vi "Read Cursors.vi"(0 "VISA Resource Name":refnum<visa-resource-name>, 11 "error in (no error)":errorcluster) -> (1 "horiz pos 1":dbl format="%.7f", 2 "horiz pos 2":dbl format="%.7f", 3 "horiz delta":dbl format="%.7f", 4 "VISA Resource Name Out":refnum<visa-resource-name>, 6 "horiz units":i32(ring) items=["Volts", "Amps", "Amp^2", "Amp/Volt", "Volt/Amp", "Volts^2", "Watt", "%", "IRE"], 10 "vert units":i32(ring) items=["Seconds", "Hertz", "Percent", "Degrees"], 12 "vert pos 1":dbl format="%.7f", 13 "vert pos 2":dbl format="%.7f", 14 "vert delta":dbl format="%.7f", 15 "error out":errorcluster)   [LabVIEW 2010, in "Tektronix TDS 3000 Series.lvlib"]
doc: "This VI returns the positions, delta values and units of the horizontal and vertical cursors on the scope."
uses:
  <instrlib>/Tektronix TDS 3000 Series/Tektronix TDS 3000 Series.lvlib
  <vilib>/Utility/error.llb/whitespace.ctl
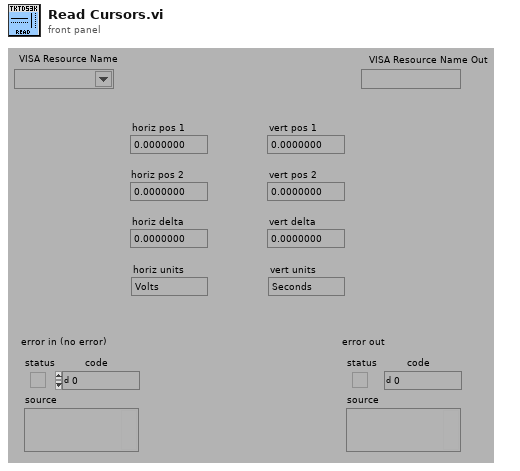
[diagram p1: front panel]
types:
  T1 = typedef "whitespace.ctl" = u16
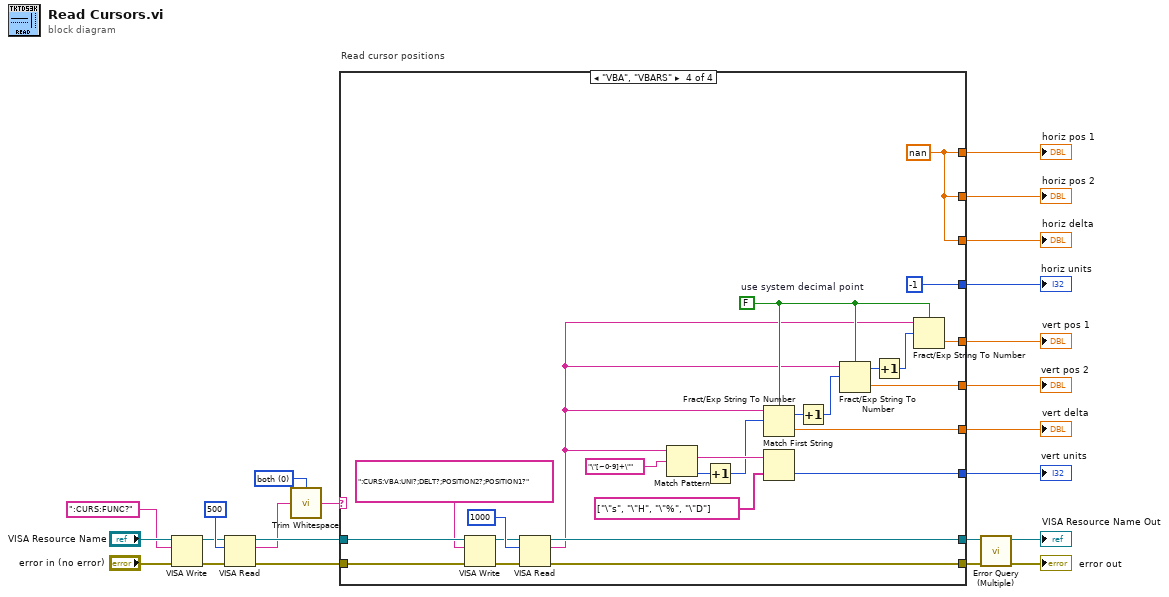
[diagram p0: block diagram]
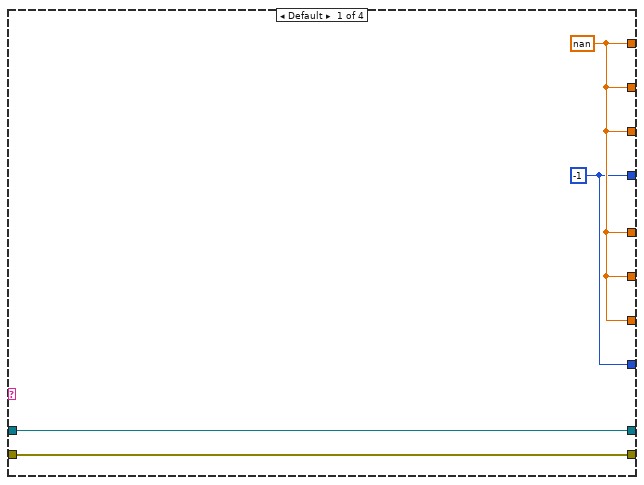
[diagram p2: hidden frame]
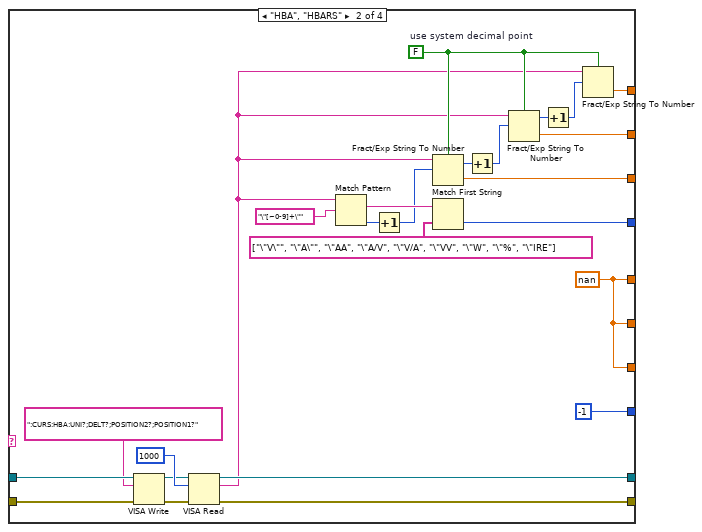
[diagram p3: hidden frame]
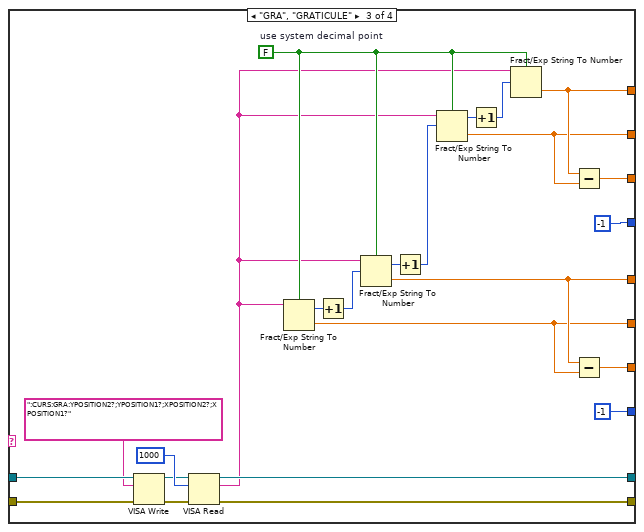
[diagram p4: hidden frame]
diagram:
  w7 = T1 0 items=["both", "start of string", "end of string"] ("location (both)")
  # "Read cursor positions"
  n1 = VISA Write(VISA resource name="VISA Resource Name", write buffer=":CURS:FUNC?", error in (no error)="error in (no error)") -> (VISA resource name out=w19:refnum<visa-resource-name>, error out=w18:errorcluster)  [unwired: 1 out]
  n2 = VISA Read(VISA resource name=w19, byte count=u32 500, error in (no error)=w18) -> (VISA resource name out=w11:refnum<visa-resource-name>, read buffer=w8:string, error out=w10:errorcluster)  [unwired: 1 out]
  n3 = call <vilib>:"Trim Whitespace.vi"("string"=w8, "location (both)"=w7) -> ("trimmed string"=w9:string)
  n4 = case shown="\"VBA\", \"VBARS\"" w9 {
    tunnel: [w25 w40 w58 w98] -> w17
    tunnel: [w25 w39 w57 w98] -> w16
    tunnel: [w25 w38 w56 w98] -> w15
    tunnel: [w25 w41 w54 w80] -> w14
    tunnel: [w25 w41 w53 w81] -> w13
    tunnel: [w25 w41 w55 w82] -> w12
    tunnel: [w26 w52 w76 w101] -> w3
    tunnel: [w27 w51 w75 w100] -> w4
    tunnel: w11 -> [w27 w48 w73 w97]
    tunnel: w10 -> [w26 w45 w70 w94]
    tunnel: [w24 -1 ("index") -1 ("index") w83] -> w6
    tunnel: [w24 w37 -1 ("index") -1 ("index")] -> w5
    frame Default {
      w24 = -1 ("index")
      w25 = nan
    }
    frame "HBA", "HBARS" {
      w49 = FALSE  # use system decimal point
      w41 = nan
      n5 = VISA Write(VISA resource name=w48, write buffer=":CURS:HBA:UNI?;DELT?;POSITION2?;POSITION1?", error in (no error)=w45) -> (VISA resource name out=w47:refnum<visa-resource-name>, error out=w46:errorcluster)  [unwired: 1 out]
      n6 = VISA Read(VISA resource name=w47, byte count=u32 1000, error in (no error)=w46) -> (VISA resource name out=w51:refnum<visa-resource-name>, read buffer=w36:string, error out=w52:errorcluster)  [unwired: 1 out]
      n7 = Match Pattern(string=w36, regular expression="\"[~0-9]+\"") -> (match substring=w31:string, offset past match=w30:i32)  [unwired: 1 in, 2 out]
      n8 = Increment(x=w30) -> (x+1=w29:i32)
      n9 = Fract/Exp String To Number(use system decimal point (T)=w49, string=w36, offset=w29) -> (offset past number=w35:i32, number=w38:dbl)  [unwired: 1 in]
      n10 = Match First String(2:string[] ["\"V\"", "\"A\"", "\"AA", "\"A/V", "\"V/A", "\"VV", "\"W", "\"%", "\"IRE"], 3:w31) -> (0:w37:i32)  [unwired: 1 out]
      n11 = Increment(x=w35) -> (x+1=w34:i32)
      n12 = Fract/Exp String To Number(use system decimal point (T)=w49, string=w36, offset=w34) -> (offset past number=w33:i32, number=w39:dbl)  [unwired: 1 in]
      n13 = Increment(x=w33) -> (x+1=w32:i32)
      n14 = Fract/Exp String To Number(use system decimal point (T)=w49, string=w36, offset=w32) -> (number=w40:dbl)  [unwired: 1 in, 1 out]
    }
    frame "GRA", "GRATICULE" {
      w60 = FALSE  # use system decimal point
      n15 = VISA Write(VISA resource name=w73, write buffer=":CURS:GRA:YPOSITION2?;YPOSITION1?;XPOSITION2?;XPOSITION1?", error in (no error)=w70) -> (VISA resource name out=w72:refnum<visa-resource-name>, error out=w71:errorcluster)  [unwired: 1 out]
      n16 = VISA Read(VISA resource name=w72, byte count=u32 1000, error in (no error)=w71) -> (VISA resource name out=w75:refnum<visa-resource-name>, read buffer=w59:string, error out=w76:errorcluster)  [unwired: 1 out]
      n17 = Fract/Exp String To Number(use system decimal point (T)=w60, string=w59) -> (offset past number=w62:i32, number=w53:dbl)  [unwired: 2 in]
      n18 = Increment(x=w62) -> (x+1=w61:i32)
      n19 = Fract/Exp String To Number(use system decimal point (T)=w60, string=w59, offset=w61) -> (offset past number=w66:i32, number=w54:dbl)  [unwired: 1 in]
      n20 = Increment(x=w66) -> (x+1=w65:i32)
      n21 = Fract/Exp String To Number(use system decimal point (T)=w60, string=w59, offset=w65) -> (offset past number=w64:i32, number=w57:dbl)  [unwired: 1 in]
      n22 = Increment(x=w64) -> (x+1=w63:i32)
      n23 = Fract/Exp String To Number(use system decimal point (T)=w60, string=w59, offset=w63) -> (number=w58:dbl)  [unwired: 1 in, 1 out]
      n24 = Subtract(x=w58, y=w57) -> (x-y=w56:dbl)
      n25 = Subtract(x=w54, y=w53) -> (x-y=w55:dbl)
    }
    frame "VBA", "VBARS" {
      w91 = FALSE  # use system decimal point
      w98 = nan
      n26 = VISA Write(VISA resource name=w97, write buffer=":CURS:VBA:UNI?;DELT?;POSITION2?;POSITION1?", error in (no error)=w94) -> (VISA resource name out=w96:refnum<visa-resource-name>, error out=w95:errorcluster)  [unwired: 1 out]
      n27 = VISA Read(VISA resource name=w96, byte count=u32 1000, error in (no error)=w95) -> (VISA resource name out=w100:refnum<visa-resource-name>, read buffer=w79:string, error out=w101:errorcluster)  [unwired: 1 out]
      n28 = Match Pattern(string=w79, regular expression="\"[~0-9]+\"") -> (match substring=w86:string, offset past match=w85:i32)  [unwired: 1 in, 2 out]
      n29 = Increment(x=w85) -> (x+1=w84:i32)
      n30 = Fract/Exp String To Number(use system decimal point (T)=w91, string=w79, offset=w84) -> (offset past number=w90:i32, number=w82:dbl)  [unwired: 1 in]
      n31 = Match First String(2:string[] ["\"s", "\"H", "\"%", "\"D"], 3:w86) -> (0:w83:i32)  [unwired: 1 out]
      n32 = Increment(x=w90) -> (x+1=w89:i32)
      n33 = Fract/Exp String To Number(use system decimal point (T)=w91, string=w79, offset=w89) -> (offset past number=w88:i32, number=w81:dbl)  [unwired: 1 in]
      n34 = Increment(x=w88) -> (x+1=w87:i32)
      n35 = Fract/Exp String To Number(use system decimal point (T)=w91, string=w79, offset=w87) -> (number=w80:dbl)  [unwired: 1 in, 1 out]
    }
  }
  "vert units" <- w6
  "horiz pos 1" <- w17
  "horiz pos 2" <- w16
  "horiz delta" <- w15
  "vert pos 1" <- w14
  "vert pos 2" <- w13
  "vert delta" <- w12
  "horiz units" <- w5
  n36 = call <instrlib>:"Error Query (Multiple).vi"("error in (no error)"=w3, "VISA Resource Name"=w4) -> ("error out"=→"error out":errorcluster, "VISA Resource Name Out"=→"VISA Resource Name Out":refnum<visa-resource-name>)  [unwired: 6 in, 2 out]
